vi "Build_Slack_text.vi"(7 "Collection Info Array":T1[](array[typedef]), 9 "Chemical":string, 10 "Scan Type":string, 11 "New Date Name":string) -> (3 "Slack String":string)   [LabVIEW 2018]
uses:
  Type defs/FileAcq_v1_Ctrl.ctl
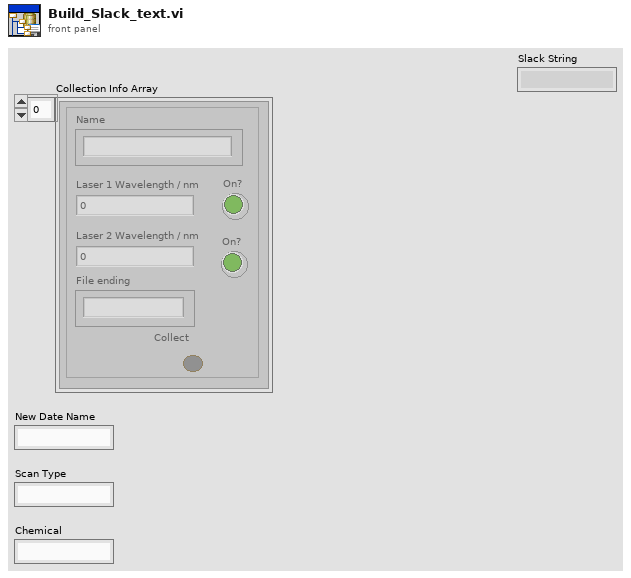
[diagram p1: front panel]
types:
  T1 = typedef "FileAcq_v1_Ctrl.ctl" = cluster{"Type":string, "LaserWave1":dbl, "Shutter1":bool, "LaserWave2":dbl, "Shutter2":bool, "FileEnd":string, "Collect":bool}
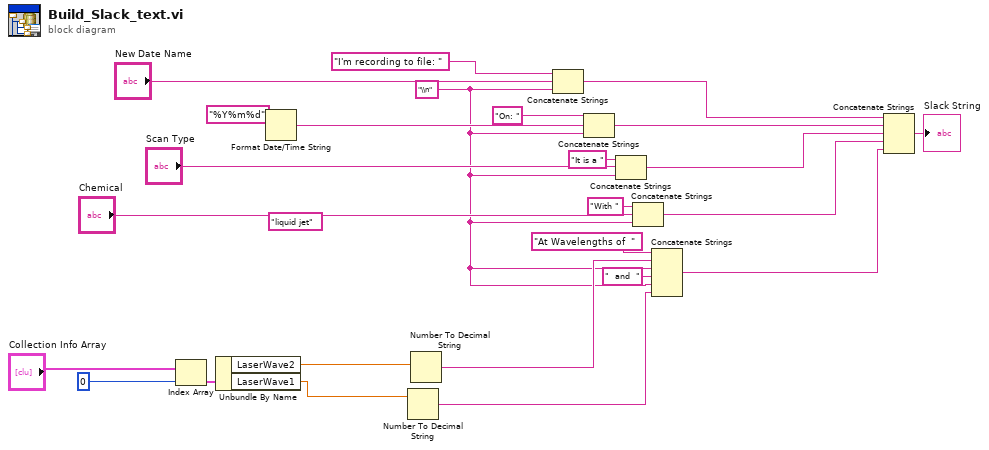
[diagram p0: block diagram]
diagram:
  w4 = "\\n" ("string")
  (unwired) "liquid jet" ("experiment")
  n1 = Index Array(array="Collection Info Array", index=0) -> (element=w24:T1)
  n2 = Unbundle By Name(w24) -> ("LaserWave2"=w25:dbl, "LaserWave1"=w3:dbl)
  n3 = Format Date/Time String(time format string (%c)="%Y%m%d") -> (date/time string=w17:string)  [unwired: 2 in]
  n4 = Number To Decimal String(number=w3) -> (decimal integer string=w2:string)  [unwired: 1 in]
  n5 = Number To Decimal String(number=w25) -> (decimal integer string=w7:string)  [unwired: 1 in]
  n6 = Concatenate Strings("I'm recording to file: " ("string"), "New Date Name", w4) -> (w16:string)
  n7 = Concatenate Strings("On: " ("string"), w17, w4) -> (w15:string)
  n8 = Concatenate Strings("It is a " ("string"), "Scan Type", w4) -> (w12:string)
  n9 = Concatenate Strings("With " ("string"), "Chemical", w4) -> (w9:string)
  n10 = Concatenate Strings("At Wavelengths of  " ("string"), w7, w4, "  and  " ("string"), w4, w2) -> (w6:string)
  n11 = Concatenate Strings(w16, w15, w12, w9, w6) -> (→"Slack String":string)
